vi "ERA_Select.vi"(8 "Error In":errorcluster, 9 "Ind_end":i32, 10 "Ind_begin":i32, 11 "Data In":waveform(dbl)[](array[waveform])) -> (0 "Error Out":errorcluster, 3 "Data Out":waveform(dbl)[](array[waveform]))   [LabVIEW 2017, in "AppPlugins.lvlib" / "EraPlugin.lvclass"]
uses:
  EraPlugin.lvclass
  <vilib>/Waveform/WDTOps.llb/WDT Get Waveform Subset DBL.vi
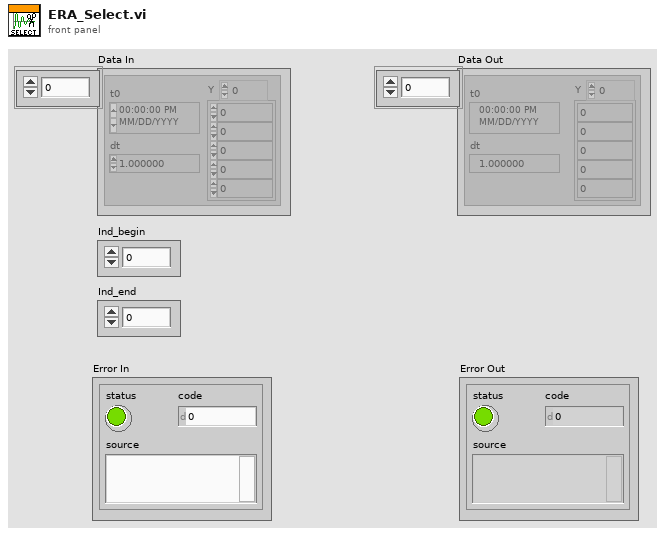
[diagram p1: front panel]
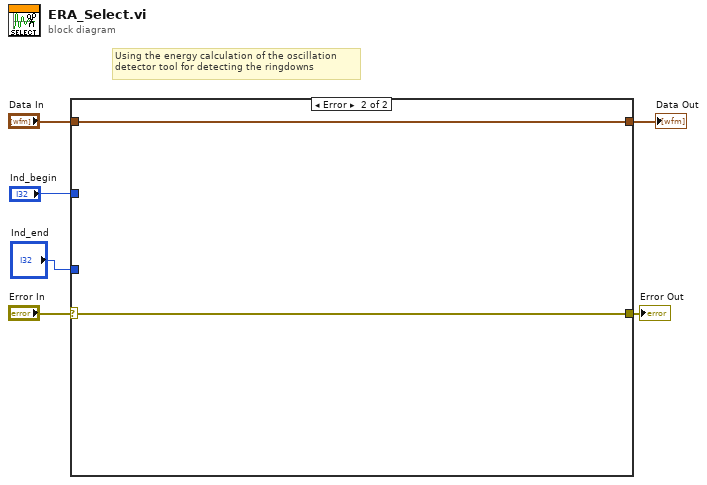
[diagram p0: block diagram]
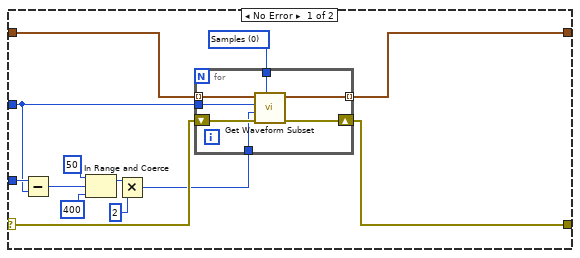
[diagram p2: hidden frame]
diagram:
  # "Using the energy calculation of the oscillation \ndetector tool for detecting the ringdowns"
  n1 = case shown="Error" "Error In" {
    selector: "Error In" -> [w16 w27]
    tunnel: "Data In" -> [w18 w28]
    tunnel: [w17 w28] -> w4
    tunnel: [w15 w27] -> w3
    tunnel: "Ind_begin" -> [w8 _]
    tunnel: "Ind_end" -> [w9 _]
    frame No Error {
      w19 = u16 0 items=["Samples", "Relative Time"] ("start/duration format")
      n2 = Subtract(x=w9, y=w8) -> (x-y=w7:i32)
      n3 = In Range and Coerce(upper limit=50, x=w7, lower limit=400) -> (coerced(x)=w12:i32)  [unwired: 1 out]
      n4 = Multiply(x=w12, y=2) -> (x*y=w10:i32)
      n5 = for {
        tunnel: [w26] -> w17 mode=indexing
        shift-right: [w25] -> w15
        shift-left: w16 -> [w24]
        tunnel: w19 -> [w23]
        tunnel: w18 -> [w22] mode=indexing
        tunnel: w8 -> [w21]
        tunnel: w10 -> [w20]
        n6 = call-poly <vilib>:"Get Waveform Subset.vi"("start/duration format"=w23, "error in (no error)"=w24, "duration"=w20, "start samples/time"=w21, "waveform in"=w22) -> ("error out"=w25:errorcluster, "waveform out"=w26:waveform(dbl))  [unwired: 1 in, 2 out]
      }
    }
    frame Error {
    }
  }
  "Data Out" <- w4
  "Error Out" <- w3
